vi "simple case.vi"() -> ()   [LabVIEW 2013, in "libusvlv.lvlib"]
uses:
  libusvlv.lvlib
  UsbCom.dll
panel:
  in  "COMMAND":u16(ring) items=["STARTBIN", "STARTDEP", "STARTBMP"]
  in  "read ep":i32=129 format="%x"
  out "file length":u32
  in  "stop":bool
  out "receive":u8[](array[numeric])
  out "recevied":bool
  out "SerialNumber":string
  out "len":i32
  in  "byte buffer":string="00000000000000000000"
  out "size":i32
  in  "wirte ep":i32=3 format="%x"
  in  "size":i32=1024 step=1024
  in  "timeout":i32=2000
  out "START send":bool
  out "usb opend":bool
  out "flag":u32
  out "altinterface":i32
  out "interface":i32
  out "configure":i32
  in  "index":i32
  in  "START":bool
  in  "vid":u32=21317 format="%x"
  in  "pid":u32=4660 format="%x"
  out "devices":u32
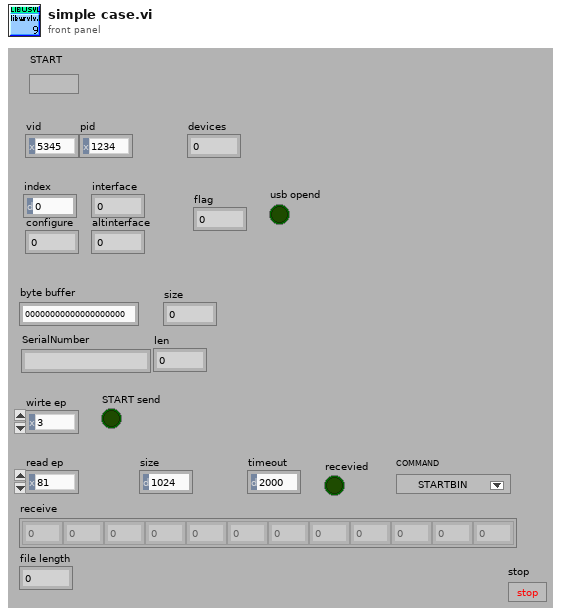
[diagram p1: front panel]
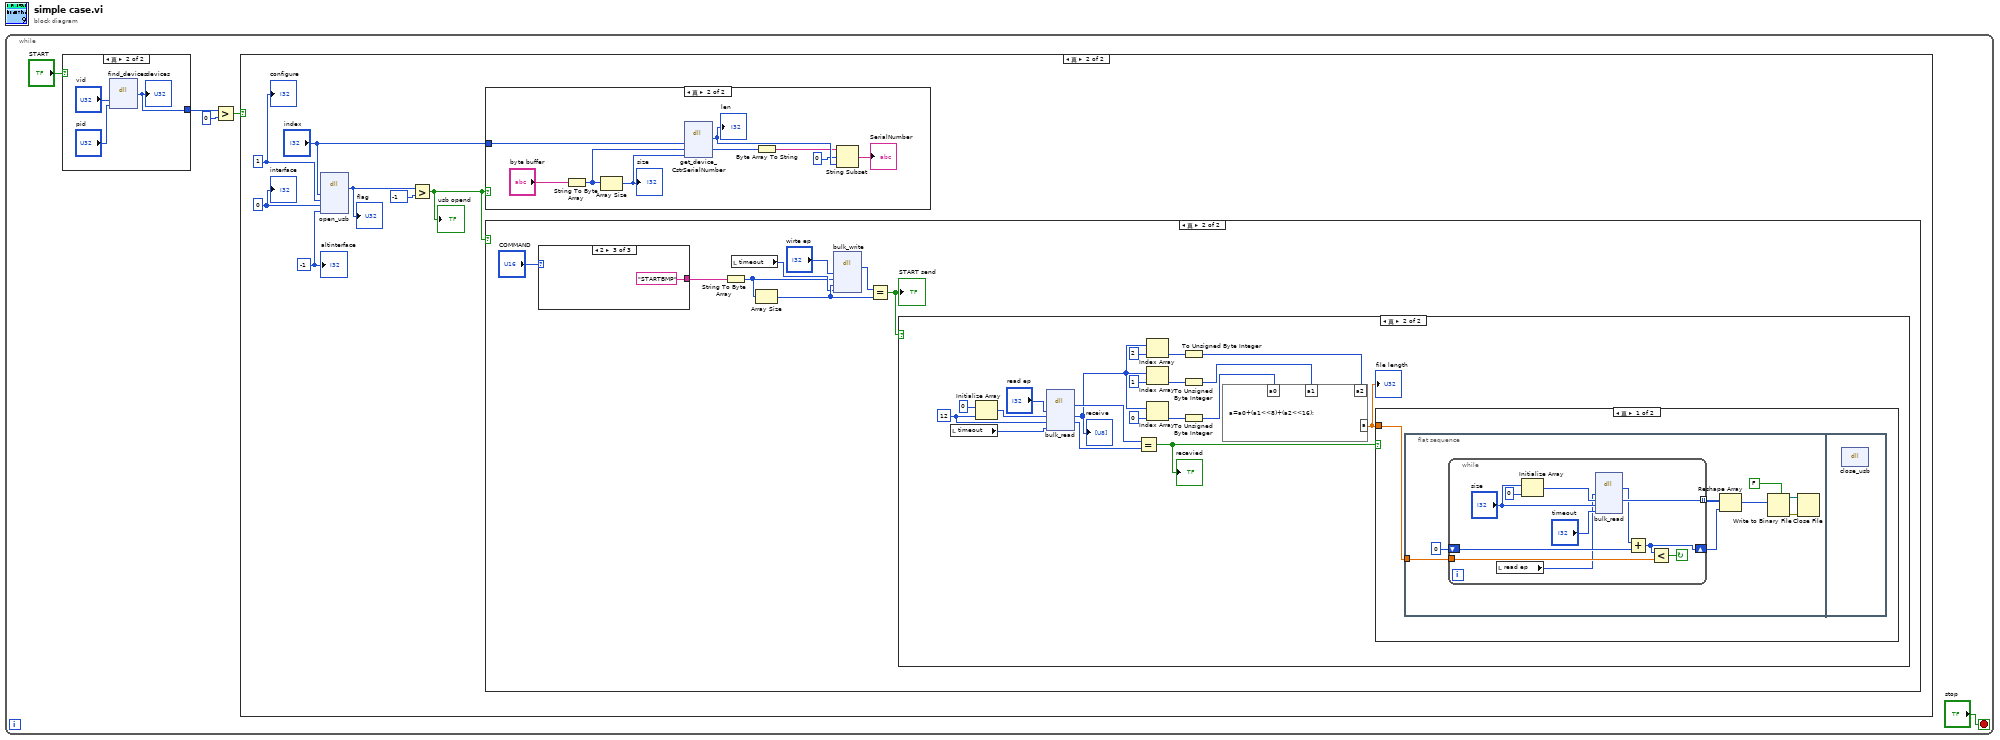
[diagram p0: block diagram]
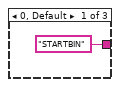
[diagram p5: hidden frame]
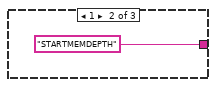
[diagram p6: hidden frame]
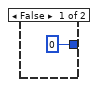
[diagram p9: hidden frame]
diagram:
  n1 = while {
    stop <- "stop" stop-if-true
    n2 = case shown="真" "START" {
      tunnel: [0 w73] -> w4
      frame False {
      }
      frame True {
        n3 = dll-call lib="E:/libusvlv/UsbCom.dll" fn="find_devices"("vid"="vid", "pid"="pid") -> ("num"=w73:i32)  [unwired: 5 in, 2 out]
        "devices" <- w73
      }
    }
    n4 = Greater?(x=w4, y=0) -> (0:w2:bool)
    n5 = case shown="真" w2 {
      frame False {
      }
      frame True {
        w7 = -1
        w8 = 0
        w9 = 1
        n6 = dll-call lib="E:/libusvlv/UsbCom.dll" fn="open_usb"("idx"="index", "conf"=w9, "iface"=w8, "altiface"=w7) -> ("返回类型"=w12:i32)  [unwired: 7 in, 2 out]
        "flag" <- w12
        n7 = Greater?(x=w12, y=-1) -> (0:w10:bool)
        "usb opend" <- w10
        n8 = case shown="真" w10 {
          tunnel: "index" -> [_ w13]
          frame False {
          }
          frame True {
            n9 = String To Byte Array(string="byte buffer") -> (unsigned byte array=w19:u8[])
            n10 = Array Size(array=w19) -> (size(s)=w20:i32)
            "size" <- w20
            n11 = dll-call lib="E:/libusvlv/UsbCom.dll" fn="get_device_CstrSerialNumber"("idx"=w13, "str"=w19, "len"=w20) -> ("size"=w17:i32, "str"=w18:i8[])  [unwired: 5 in, 2 out]
            "len" <- w17
            n12 = Byte Array To String(unsigned byte array=w18) -> (string=w15:string)
            n13 = String Subset(string=w15, offset (0)=0, length (rest)=w17) -> (substring=→"SerialNumber":string)
          }
        }
        n14 = case shown="真" w10 {
          frame False {
          }
          frame True {
            n15 = case shown="2" "COMMAND" {
              tunnel: ["STARTBIN" "STARTMEMDEPTH" "STARTBMP"] -> w22
              frame 0, Default {
              }
              frame 1 {
              }
              frame 2 {
              }
            }
            n16 = String To Byte Array(string=w22) -> (unsigned byte array=w24:u8[])
            n17 = local read "timeout"() -> (w25:i32)
            n18 = Array Size(array=w24) -> (size(s)=w27:i32)
            n19 = dll-call lib="E:/libusvlv/UsbCom.dll" fn="bulk_write"("ep"="wirte ep", "bytes"=w24, "size"=w27, "timeout"=w25) -> ("size"=w28:i32)  [unwired: 6 in, 3 out]
            n20 = Equal?(x=w28, y=w27) -> (x = y?=w29:bool)
            "START send" <- w29
            n21 = case shown="真" w29 {
              frame False {
              }
              frame True {
                w48 = 12
                n22 = local read "timeout"() -> (w34:i32)
                n23 = Initialize Array(0, w48) -> (w50:i32[])
                n24 = dll-call lib="E:/libusvlv/UsbCom.dll" fn="bulk_read"("ep"="read ep", "bytes"=w50, "size"=w48, "timeout"=w34) -> ("返回类型"=w49:i32, "bytes"=w46:i8[], "size"=w33:i32)  [unwired: 5 in, 2 out]
                "receive" <- w46
                n25 = Equal?(x=w49, y=w33) -> (x = y?=w47:bool)
                "recevied" <- w47
                n26 = Index Array(array=w46, index=2) -> (element=w38:i8)
                n27 = Index Array(array=w46, index=1) -> (element=w40:i8)
                n28 = Index Array(array=w46, index=0) -> (element=w42:i8)
                n29 = To Unsigned Byte Integer(number=w38) -> (unsigned 8bit integer=w37:u8)
                n30 = To Unsigned Byte Integer(number=w40) -> (unsigned 8bit integer=w39:u8)
                n31 = To Unsigned Byte Integer(number=w42) -> (unsigned 8bit integer=w41:u8)
                n32 = formula code="a=a0+(a1<<8)+(a2<<16);"("a0"=w41, "a1"=w39, "a2"=w37) -> ("a"=w36:dbl)
                "file length" <- w36
                n33 = case shown="真" w47 {
                  tunnel: w36 -> [w52 _]
                  frame True {
                    n34 = flat-sequence {
                      tunnel: w52 -> [w58]
                      frame #0 {
                        n35 = while {
                          shift-right: [w63] -> w53
                          shift-left: 0 -> [w66]
                          tunnel: [w68] -> w55 mode=indexing
                          tunnel: w58 -> [w64]
                          stop <- w65 continue-if-true
                          n36 = local read "read ep"() -> (w61:i32)
                          n37 = Initialize Array("size", 0) -> (w70:i32[])
                          n38 = dll-call lib="E:/libusvlv/UsbCom.dll" fn="bulk_read"("ep"=w61, "bytes"=w70, "size"="size", "timeout"="timeout") -> ("返回类型"=w67:i32, "bytes"=w68:i8[])  [unwired: 6 in, 2 out]
                          n39 = Add(x=w67, y=w66) -> (x+y=w63:i32)
                          n40 = Less?(x=w63, y=w64) -> (x < y?=w65:bool)
                        }
                        n41 = Reshape Array(w55, w53) -> (w54:i8[])
                        n42 = Write to Binary File(data=w54, 5:FALSE) -> (refnum out=w60:refnum<file>, error out=w59:errorcluster)  [unwired: 1 in, 4 out]
                        n43 = Close File(refnum=w60, error in=w59) -> ()  [unwired: 2 out]
                      }
                      frame #1 {
                        n44 = dll-call lib="E:/libusvlv/UsbCom.dll" fn="close_usb"() -> ()  [unwired: 3 in, 3 out]
                      }
                    }
                  }
                  frame False {
                  }
                }
              }
            }
          }
        }
        "configure" <- w9
        "interface" <- w8
        "altinterface" <- w7
      }
    }
  }
